vi "Destroy.vi"(8 "error in (no error)":errorcluster, 11 "Queue Sink in":refnum<class "Queue Sink.lvclass">) -> (0 "error out":errorcluster)   [LabVIEW 2020, in "LV Log.lvlib" / "Queue Sink.lvclass"]
uses:
  Queue Sink.lvclass
  Queue Sink.lvclass/Queue Sink.ctl
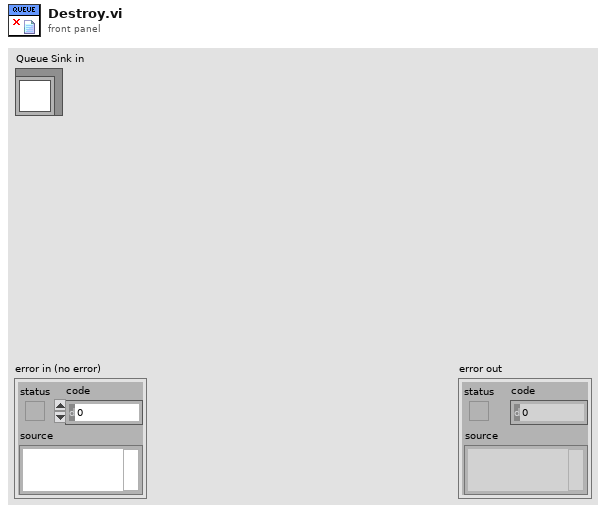
[diagram p1: front panel]
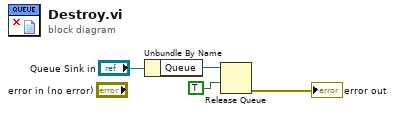
[diagram p0: block diagram]
diagram:
  n1 = Unbundle By Name("Queue Sink in") -> ("Queue"=w3:refnum<queue>)
  n2 = Release Queue(queue=w3, force destroy? (F)=TRUE) -> (error out=→"error out":errorcluster)  [unwired: 1 in, 2 out]
